vi "poseSubscriber.vi"() -> ()   [LabVIEW 2014]
uses:
  <vilib>/Tufts CEEO ROS for LabVIEW Software/ROS/Code/Console/Servers/ServerSubs/TopicDef.ctl
  <vilib>/Tufts CEEO ROS for LabVIEW Software/ROS/Code/SubVIs/_ROSDirection.ctl
panel:
  out "PoseStamped":T1
  out "I heard:":string
  out "error out":errorcluster
  in  "stop":bool
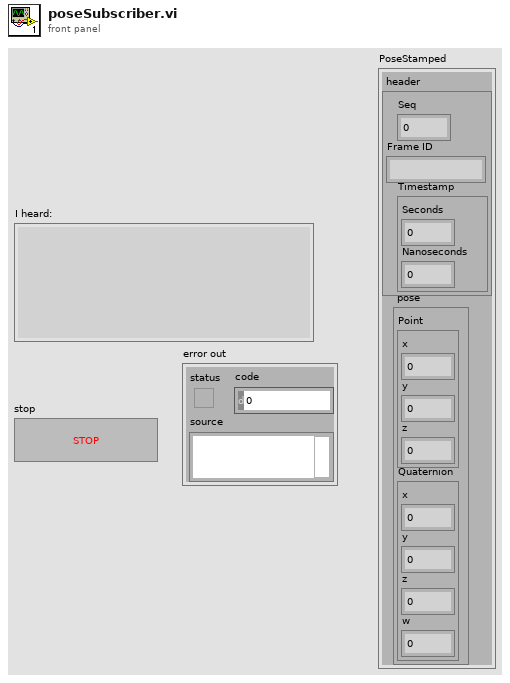
[diagram p1: front panel]
types:
  T1 = cluster{" header":cluster{"Seq":u32, "Frame ID":string, "Timestamp":cluster{"Seconds":i32, "Nanoseconds":i32}}, " pose":cluster{"Point":cluster{"x":dbl, "y":dbl, "z":dbl}, "Quaternion":cluster{"x":dbl, "y":dbl, "z":dbl, "w":dbl}}}
  T2 = typedef "TopicDef.ctl" = cluster{"Topic":string, "Type":string, "Action":T3, "Update (ms)":u16, "queue size":u16}
  T3 = typedef "_ROSDirection.ctl" = enum16{"Node", "Publisher", "Subscriber", "ServiceClient", "ServiceProvider"}
  T4 = typedef "_ROSControl.ctl" = cluster{"topic port":u16, "Node":string, "topic":string, "type":string, "node port":u16, "error ":errorcluster, "Direction":T3, "Update (ms)":u16, "FIFO size":u16}
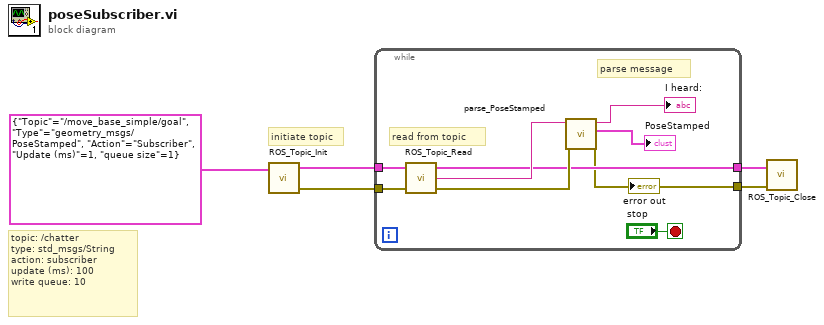
[diagram p0: block diagram]
diagram:
  # "initiate topic"
  # "topic: /chatter\ntype: std_msgs/String\naction: subscriber\nupdate (ms): 100\nwrite queue: 10"
  n1 = call <vilib>:"ROS_Topic_Init.vi"("Definitions"=T2 {"Topic"="/move_base_simple/goal", "Type"="geometry_msgs/PoseStamped", "Action"=enum."Subscriber", "Update (ms)"=1, "queue size"=1}) -> ("ROS out"=w5:T4, "error out"=w4:errorcluster)  [unwired: 2 in]
  n2 = while {
    tunnel: w5 -> [w14]
    tunnel: w4 -> [w11]
    tunnel: [w8] -> w3
    tunnel: [w7] -> w2
    stop <- "stop" stop-if-true
    # "parse message"
    # "read from topic"
    n3 = call <vilib>:"ROS_Topic_Read.vi"("error in (no error)"=w11, "ROS in"=w14) -> ("error out"=w10:errorcluster, "Reply"=w13:string, "ROS out"=w8:T4)  [unwired: 1 in]
    n4 = call <userlib>:"parse_PoseStamped.vi"("error in"=w10, "msg in"=w13) -> ("error out"=w7:errorcluster, "PoseStamped"=→"PoseStamped":T1, "msg out"=→"I heard:":string)  [unwired: 7 in]
    "error out" <- w7
  }
  n5 = call <vilib>:"ROS_Topic_Close.vi"("error in"=w2, "ROS in"=w3) -> ()  [unwired: 2 in, 1 out]
